vi "Divisor_Sum_Engine_Method_2.vi"(11 "N":i32) -> (2 "Numeric":i32, 3 "Array":i32[](array[numeric]))   [LabVIEW 2026]
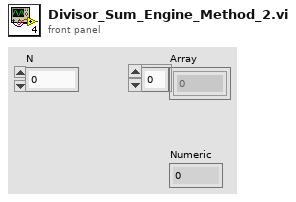
[diagram p1: front panel]
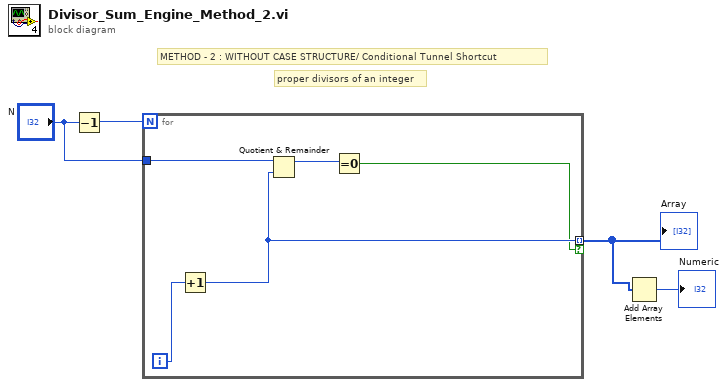
[diagram p0: block diagram]
diagram:
  # "METHOD - 2 : WITHOUT CASE STRUCTURE/ Conditional Tunnel Shortcut"
  # "proper divisors of an integer"
  n1 = Decrement(x="N") -> (x-1=w1:i32)
  n2 = for {
    N: w1 -> [_]
    tunnel: "N" -> [w8]
    tunnel: [w6] -> w3 mode=indexing if=w5
    i -> [w9]
    n3 = Increment(x=w9) -> (x+1=w6:i32)
    n4 = Quotient & Remainder(x=w8, y=w6) -> (x-y*floor(x/y)=w7:i32)  [unwired: 1 out]
    n5 = Equal To 0?(x=w7) -> (x = 0?=w5:bool)
  }
  "Array" <- w3
  n6 = Add Array Elements(numeric array=w3) -> (sum=→"Numeric":i32)
